vi "Is Data Ready.vi"(8 "error in (no error)":errorcluster) -> (0 "error out":errorcluster, 3 "function return":i32)   [LabVIEW 2023, in "vmmsolib.lvlib"]
doc: "DLL_API int WINAPI IsDataReady();"
uses:
  vmmsolib.lvlib
  vmmso.dll
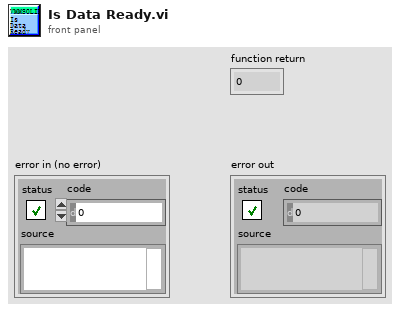
[diagram p1: front panel]
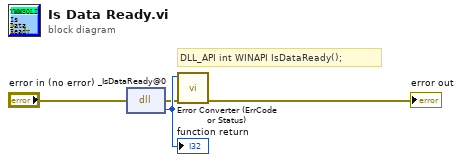
[diagram p0: block diagram]
diagram:
  # "DLL_API int WINAPI IsDataReady();"
  n1 = dll-call lib="D:/VmMsoSDK/demo-Labview/2023/vmmsolib/vmmso.*" fn="_IsDataReady@0"(error in="error in (no error)") -> (error out=w2:errorcluster, w4:i32)  [unwired: 2 in, 1 out]
  "function return" <- w4
  n2 = call "Error Converter (ErrCode or Status).vi"("error in (no error)"=w2, "error code"=w4) -> ("error out"=→"error out":errorcluster)  [unwired: 9 in]
